vi "interface.vi"() -> ()   [LabVIEW 2019]
panel:
  out "naar volgende  index":bool
  in  "af te leggen route":dbl[](array[numeric])
  out "lijndetectie":dbl[](array[numeric])
  out "groen":bool
  in  "achteruit":bool
  in  "rechtdoor":bool
  in  "rechts":bool
  in  "links":bool
  in  "manueel":bool
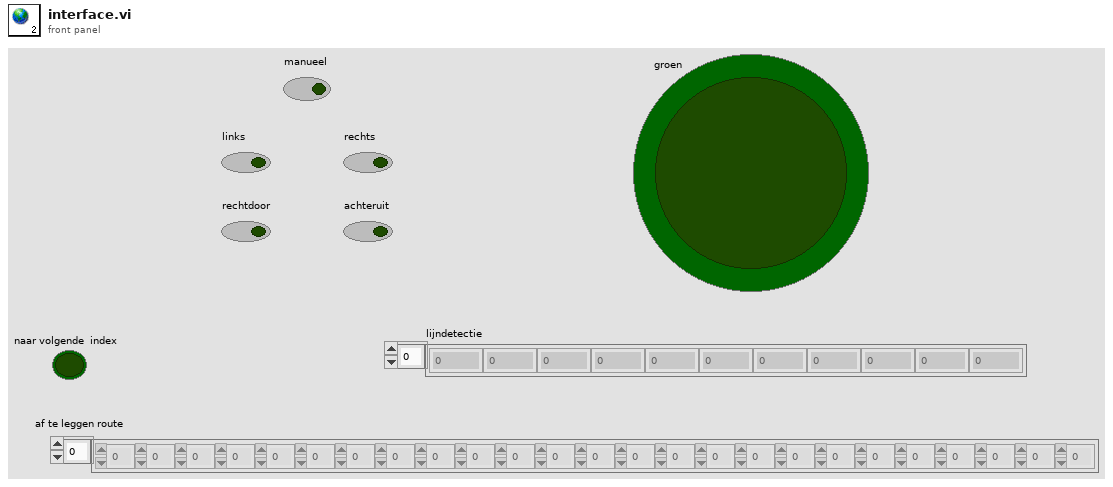
[diagram p1: front panel]
diagram:
